vi "Exchange Param.vi"(8 "error in (no error)":errorcluster, 9 "PAR":dbl[](array[numeric]), 10 "AOP":dbl[][](array[numeric]), 11 "Regs":refnum<class "bronkhorst_reg_2.lvclass">[](array[class])) -> (0 "error out":errorcluster, 3 "Regs out":refnum<class "bronkhorst_reg_2.lvclass">[](array[class]))   [LabVIEW 2019, in "control.lvlib" / "bronkhorst_reg_2.lvclass"]
uses:
  bronkhorst_reg_2.lvclass
  D:/my_projects/projects/Algorithms/Labview/19/Reg/Y_Limiter/Y_Limiter.lvclass
  bronkhorst_reg_2.lvclass/bronkhorst_reg_2.ctl
  Inputs/Ctl/AOParamColumns.ctl
  Y_Limiter/Y_Limiter.lvclass/Y_Limiter.ctl
  Inputs/Inputs.lvlib
  Y_Limiter/Y_Limiter.lvclass
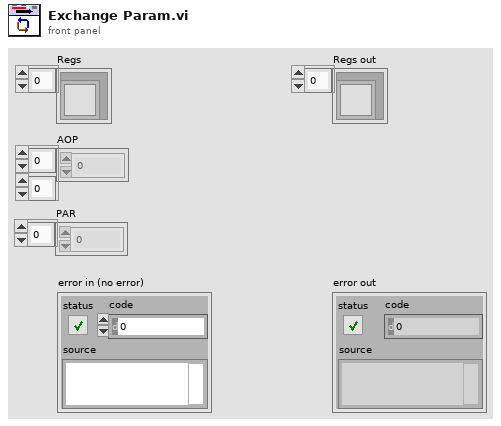
[diagram p1: front panel]
types:
  T1 = typedef "Inputs.lvlib/AOParamColumns.ctl" = enum16{"instrument_gain", "instrument_offset", "instrument_range_min", "instrument_range_max", "output_pv_min", "output_pv_max", "output_register_min", "output_register_max", "module_fcode_full", "control_channel_num", "fcode", "fcodef", "fcode_full", "fname", "instrument_units"}
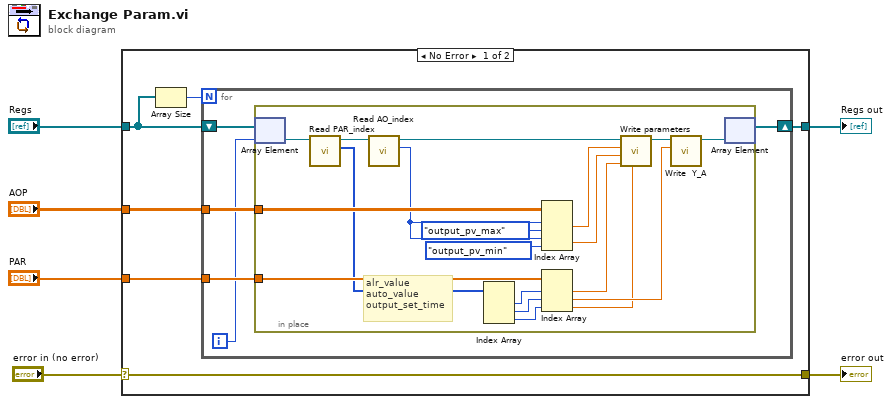
[diagram p0: block diagram]
diagram:
  n1 = case shown="No Error" "error in (no error)" {
    selector: "error in (no error)" -> [w7 w38]
    tunnel: [w12 w37] -> w6
    tunnel: "AOP" -> [w11 _]
    tunnel: "PAR" -> [w10 _]
    tunnel: "Regs" -> [w8 w37]
    tunnel: [w7 w38] -> w1
    frame No Error {
      n2 = Array Size(array=w8) -> (size(s)=w9:i32)
      n3 = for {
        N: w9 -> [_]
        tunnel: w11 -> [w17]
        tunnel: w10 -> [w16]
        shift-right: [w13] -> w12
        shift-left: w8 -> [w15]
        i -> [w14]
        n4 = in-place {
          in-place-border: w17 -> [w36]
          in-place-border: w16 -> [w35]
          # "alr_value\nauto_value\noutput_set_time"
          n5 = in-place-array #1(w15, w14) -> (w29:refnum<class "bronkhorst_reg_2.lvclass">)
          n6 = call "Read PAR_index.vi"("bronkhorst_reg in"=w29) -> ("PAR_indexes"=w21:i32[], "bronkhorst_reg out"=w30:refnum<class "bronkhorst_reg_2.lvclass">)  [unwired: 9 in]
          n7 = call "Read AO_index.vi"("bronkhorst_reg in"=w30) -> ("AO_index"=w31:i32, "bronkhorst_reg out"=w27:refnum<class "bronkhorst_reg_2.lvclass">)  [unwired: 9 in]
          n8 = Index Array(array=w21) -> (element #1=w20:i32, element #2=w19:i32, element #3=w18:i32)  [unwired: 3 in]
          n9 = Index Array(array=w36, index (row) #1=w31, index (col) #1=AOParamColumns."output_pv_max" ("AOParamColumns"), index (row) #2=w31, index (col) #2=AOParamColumns."output_pv_min" ("AOParamColumns")) -> (element #1=w26:dbl, element #2=w25:dbl)
          n10 = Index Array(array=w35, index #1=w20, index #2=w19, index #3=w18) -> (element #1=w24:dbl, element #2=w32:dbl, element #3=w23:dbl)
          n11 = call "Write parameters.vi"("output set time"=w23, "alr value"=w24, "output L"=w25, "output H"=w26, "Y_Limiter in"=w27) -> ("Y_Limiter out"=w22:refnum<class "bronkhorst_reg_2.lvclass">)  [unwired: 6 in]
          n12 = call "Write  Y_A.vi"("Y_A"=w32, "reg in"=w22) -> ("reg out"=w28:refnum<class "bronkhorst_reg_2.lvclass">)  [unwired: 9 in]
          n13 = in-place-array #1(w28) -> (w13:refnum<class "bronkhorst_reg_2.lvclass">[])  [unwired: 1 out]
        }
      }
    }
    frame Error {
    }
  }
  "Regs out" <- w6
  "error out" <- w1
